vi "Prototype.vi"(8 "error in (no error)":errorcluster, 11 "Message Scripter in":refnum<class "Message Scripter.lvclass">) -> (0 "error out":errorcluster, 3 "Message Scripter out":refnum<class "Message Scripter.lvclass">)   [LabVIEW 2020, in "Message Maker.lvlib" / "Message Scripter.lvclass"]
uses:
  Message Scripter.lvclass
  Message Scripter.lvclass/Message Scripter.ctl
  Prototyper/Prototyper.lvclass
  <vilib>/ErrorRing/Error Ring.xnode
  <vilib>/Utility/error.llb/Error Cluster From Error Code.vi
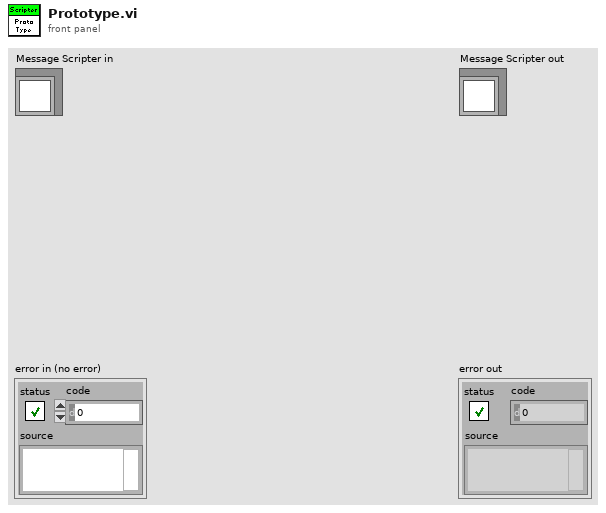
[diagram p1: front panel]
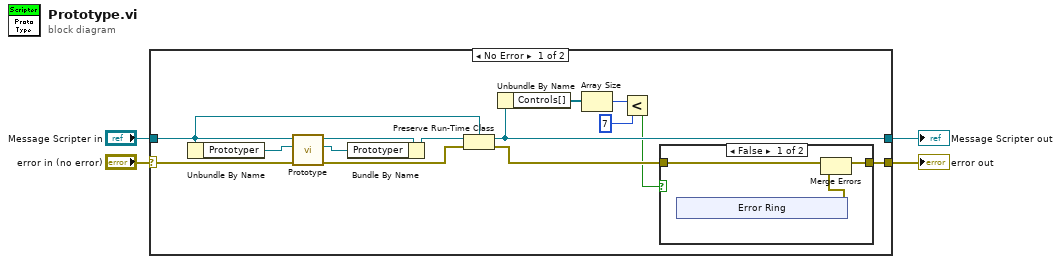
[diagram p0: block diagram]
diagram:
  n1 = case shown="No Error" "error in (no error)" {
    selector: "error in (no error)" -> [w12 w29]
    tunnel: [w7 w29] -> w3
    tunnel: [w11 w28] -> w1
    tunnel: "Message Scripter in" -> [w14 w28]
    frame No Error {
      n2 = Unbundle By Name(w14) -> ("Prototyper"=w17:refnum<class "Prototyper.lvclass">)
      n3 = call-dynamic "Prototype.vi"("error in (no error)"=w12, "Prototyper in"=w17, "Scripter in"=w14) -> ("error out"=w13:errorcluster, "Prototyper out"=w16:refnum<class "Prototyper.lvclass">, "Scripter out"=w18:refnum<class "Message Scripter.lvclass">)  [unwired: 6 in]
      n4 = Bundle By Name(cluster=w18, "Prototyper"=w16) -> (w15:refnum<class "Message Scripter.lvclass">)
      n5 = Preserve Run-Time Class(object in=w15, error in=w13, 2:w14) -> (object out=w11:refnum<class "Message Scripter.lvclass">, error out=w6:errorcluster)
      n6 = Unbundle By Name(w11) -> ("Controls[]"=w9:refnum<vi>[])
      n7 = Array Size(array=w9) -> (size(s)=w10:i32)
      n8 = Less?(x=w10, y=7) -> (x < y?=w5:bool)
      n9 = case shown="False" w5 {
        tunnel: [w20 w27] -> w7
        tunnel: w6 -> [w21 w27]
        frame False {
          n10 = xnode "Error Ring"() -> ("error out"=w19:errorcluster)
          n11 = Merge Errors(w21, w19) -> (w20:errorcluster)
        }
        frame True {
        }
      }
    }
    frame Error {
    }
  }
  "error out" <- w3
  "Message Scripter out" <- w1
